vi "_Baes64 To Doubles.vi"(1 "Little Endian (F)":bool, 2 "Base64 String":string) -> (0 "Doubles":dbl[](array[numeric]) format="%#.6f")   [LabVIEW 2012]
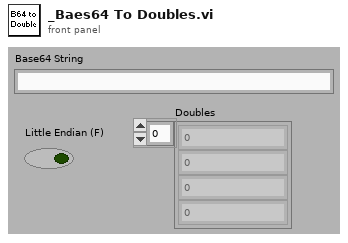
[diagram p1: front panel]
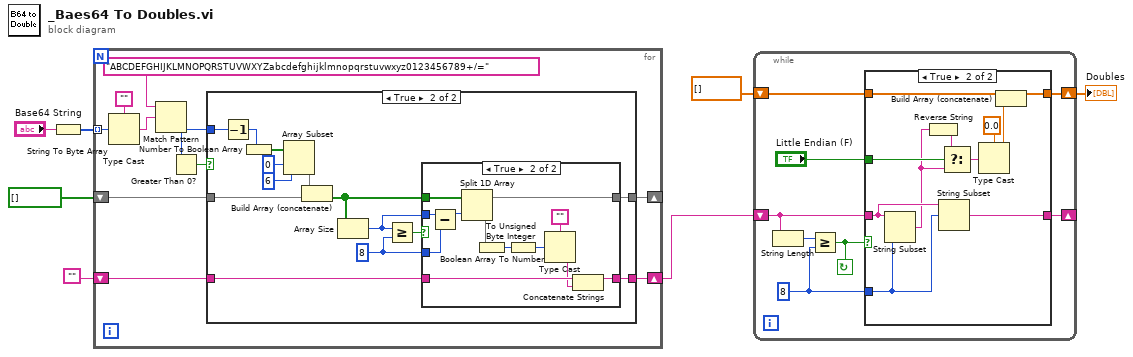
[diagram p0: block diagram]
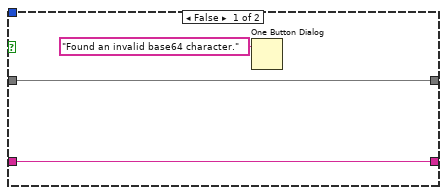
[diagram p3: hidden frame]
diagram:
  n1 = String To Byte Array(string="Base64 String") -> (unsigned byte array=w6:u8[])
  n2 = for {
    tunnel: w6 -> [w17] mode=indexing
    shift-right: [w12] -> _
    shift-left: bool[] [] -> [w13]
    shift-right: [w10] -> w4
    shift-left: "" -> [w11]
    n3 = Type Cast(type="", x=w17) -> (*(type *) &x=w14:string)
    n4 = Match Pattern(string="ABCDEFGHIJKLMNOPQRSTUVWXYZabcdefghijklmnopqrstuvwxyz0123456789+/=", regular expression=w14) -> (offset past match=w8:i32)  [unwired: 1 in, 3 out]
    n5 = Greater Than 0?(x=w8) -> (x > 0?=w9:bool)
    n6 = case shown="True" w9 {
      tunnel: w8 -> [_ w34]
      tunnel: w13 -> [w19 w28]
      tunnel: [w19 w25] -> w12
      tunnel: w11 -> [w18 w22]
      tunnel: [w18 w21] -> w10
      frame False {
        n7 = One Button Dialog(message="Found an invalid base64 character.") -> ()  [unwired: 1 in, 1 out]
      }
      frame True {
        w24 = 8 ("Precision (32)")
        n8 = Decrement(x=w34) -> (x-1=w33:i32)
        n9 = Number To Boolean Array(number=w33) -> (Boolean array=w32:bool[])
        n10 = Array Subset(array=w32, index=0, length=6) -> (w29:bool[])
        n11 = Build Array (concatenate)(w29, w28) -> (w26:bool[])
        n12 = Array Size(array=w26) -> (size(s)=w23:i32)
        n13 = Greater Or Equal?(x=w23, y=w24) -> (x >= y?=w27:bool)
        n14 = case shown="True" w27 {
          tunnel: w26 -> [w36 w48]
          tunnel: [w36 w44] -> w25
          tunnel: w24 -> [_ w46]
          tunnel: w23 -> [_ w47]
          tunnel: w22 -> [w35 w42]
          tunnel: [w35 w41] -> w21
          frame False {
          }
          frame True {
            n15 = Subtract(x=w47, y=w46) -> (x-y=w45:i32)
            n16 = Split 1D Array(array=w48, index=w45) -> (first subarray=w44:bool[], second subarray=w43:bool[])
            n17 = Boolean Array To Number(Boolean array=w43) -> (number=w39:u32)
            n18 = To Unsigned Byte Integer(number=w39) -> (unsigned 8bit integer=w37:u8)
            n19 = Type Cast(type="", x=w37) -> (*(type *) &x=w38:string)
            n20 = Concatenate Strings(w42, w38) -> (w41:string)
          }
        }
      }
    }
  }
  n21 = while {
    shift-right: [w53] -> _
    shift-left: w4 -> [w54]
    shift-right: [w49] -> w1
    shift-left: dbl[] [] -> [w50]
    stop <- w55 continue-if-true
    w52 = 8 ("Precision (32)")
    n22 = String Length(string=w54) -> (length=w56:i32)
    n23 = Greater Or Equal?(x=w56, y=w52) -> (x >= y?=w55:bool)
    n24 = case shown="True" w55 {
      tunnel: w54 -> [w58 w68]
      tunnel: [w58 w69] -> w53
      tunnel: w52 -> [_ w67]
      tunnel: "Little Endian (F)" -> [_ w66]
      tunnel: w50 -> [w57 w61]
      tunnel: [w57 w59] -> w49
      frame False {
      }
      frame True {
        n25 = String Subset(string=w68, length (rest)=w67) -> (substring=w64:string)  [unwired: 1 in]
        n26 = Reverse String(1:w64) -> (0:w65:string)
        n27 = String Subset(string=w68, offset (0)=w67) -> (substring=w69:string)  [unwired: 1 in]
        n28 = Select(t=w65, s=w66, f=w64) -> (s? t:f=w63:string)
        n29 = Type Cast(type=0.0, x=w63) -> (*(type *) &x=w60:dbl)
        n30 = Build Array (concatenate)(w61, w60) -> (w59:dbl[])
      }
    }
  }
  "Doubles" <- w1
